vi "Window-Export cam snippets.vi"(11 "Min cursor":i32) -> ()   [LabVIEW 2020]
uses:
  Functional Imaging Viewer/Typedefs/Get-Set-Clear Control.ctl
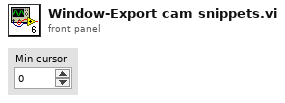
[diagram p1: front panel]
types:
  T1 = typedef "Get-Set-Clear Control.ctl" = enum16{"Get", "Set", "Clear"}
  T2 = typedef "Cam videos cluster.ctl" = cluster{"Vid 1":T3, "Vid 2":T3, "Vid 3":T3, "Vid 4":T3, "Vid1 Rel time (ms)":u32, "Vid2 Rel time (ms)":u32, "Vid3 Rel time (ms)":u32, "Vid4 Rel time (ms)":u32}
  T3 = typedef "IMAQ Image.ctl" = refnum<image>
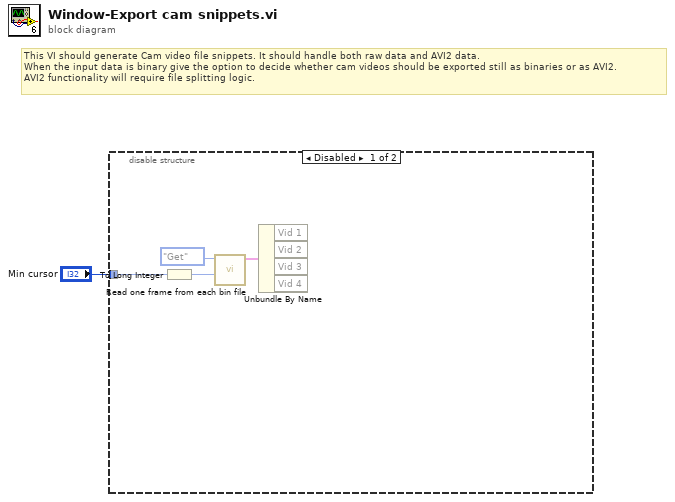
[diagram p0: block diagram]
diagram:
  # "This VI should generate Cam video file snippets. It should handle both raw data and AVI2 data.\nWhen the input data is binary give the option to decide whether cam videos should be exported still as binaries or as AVI2.\nAVI2 functionality will require file splitting logic."
  n1 = disable-structure shown="Disabled" {
    disable-tunnel: "Min cursor" -> [w5 _]
    frame Disabled {
      n2 = To Long Integer(number=w5) -> (32bit integer=w3:i32)
      n3 = call "Read one frame from each bin file.vi"("Master video's frame number (unity-based)"=w3, "Get/set"=Get-Set-Clear_Control."Get" ("GEt set .bin refs")) -> ("Cam videos cluster"=w4:T2)  [unwired: 8 in, 1 out]
      n4 = Unbundle By Name(w4) -> ()  [unwired: 4 out]
    }
    frame Enabled {
    }
  }
